vi "sensitivity (yzb).vi"(7 "sense":bool, 8 "error in (no error)":errorcluster, 11 "VISA resource name":refnum<visa-resource-name>="GPIB0::8::INSTR") -> (0 "error out":errorcluster, 5 "Sensitivity":i16(ring)=-1 items=["Auto Gain"=-1, "2 nV/fA"=0, "5 nV/fA"=1, "10 nV/fA"=2, "20 nV/fA"=3, "50 nV/fA"=4, "100 nV/fA"=5, "200 nV/fA"=6, "500 nV/fA"=7, "1 uV/pA"=8, "2 uV/pA"=9, "5 uV/pA"=10, "10 uV/pA"=11, "20 uV/pA"=12, "50 uV/pA"=13, "100 uV/pA"=14, "200 uV/pA"=15, "500 uV/pA"=16, "1 mV/nA"=17, "2 mV/nA"=18, "5 mV/nA"=19, "10 mV/nA"=20, "20 mV/nA"=21, "50 mV/nA"=22, "100 mV/nA"=23, "200 mV/nA"=24, "500 mV/mA"=25, "1 V/uA"=26])   [LabVIEW 2017]
uses:
  <vilib>/Analysis/NI_AALBase.lvlib
panel:
  out "Array":dbl[](array[numeric])
  out "Numeric":i32
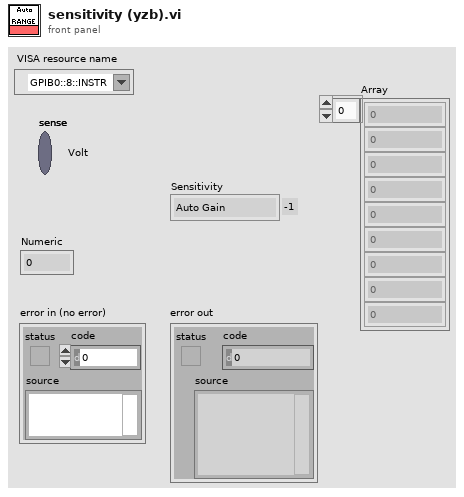
[diagram p1: front panel]
types:
  T1 = cluster{"X-Value":dbl, "Y-Value":dbl, "R-Value":dbl, "Theta-Value":dbl, "Channel 1 Display":dbl, "Channel 2 Display":dbl}
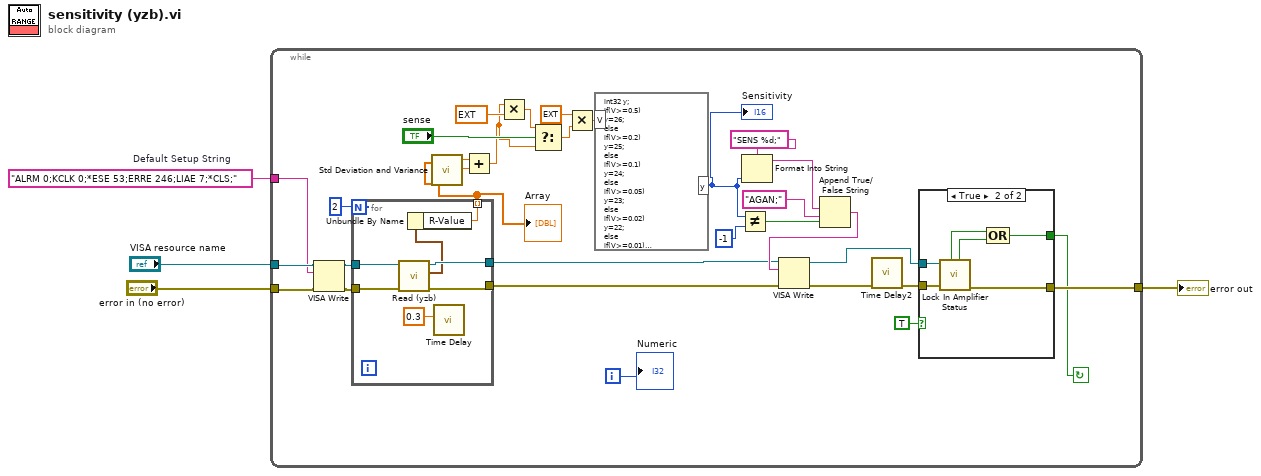
[diagram p0: block diagram]
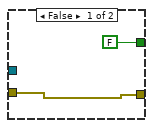
[diagram p2: hidden frame]
diagram:
  w2 = "ALRM 0;KCLK 0;*ESE 53;ERRE 246;LIAE 7;*CLS;"  # Default Setup String
  n1 = while {
    tunnel: "VISA resource name" -> [w24]
    tunnel: [w27] -> w1
    tunnel: "error in (no error)" -> [w26]
    tunnel: w2 -> [w22]
    i -> [w36]
    stop <- w17 continue-if-true
    n2 = VISA Write(VISA resource name=w24, write buffer=w22, error in (no error)=w26) -> (VISA resource name out=w23:refnum<visa-resource-name>, error out=w25:errorcluster)  [unwired: 1 out]
    n3 = for {
      N: 2 -> [_]
      tunnel: w23 -> [w51]
      tunnel: w25 -> [w50]
      tunnel: [w48] -> w19
      tunnel: [w49] -> w8 mode=indexing
      tunnel: [w46] -> w18
      n4 = call "Read (yzb).vi"("error in (no error)"=w50, "VISA resource name"=w51) -> ("error out"=w46:errorcluster, "Parameter Values"=w47:T1, "VISA resource name out"=w48:refnum<visa-resource-name>)  [unwired: 7 in]
      n5 = Unbundle By Name(w47) -> ("R-Value"=w49:dbl)
      n6 = call "Time Delay"("Delay Time (s)"=0.3) -> ()  [unwired: 10 in, 1 out]
    }
    "Array" <- w8
    n7 = call <vilib>:"Std Deviation and Variance.vi"("X"=w8) -> ("mean"=w7:dbl, "standard deviation"=w6:dbl)  [unwired: 1 in, 1 out]
    n8 = Add(x=w7, y=w6) -> (x+y=w5:dbl)
    n9 = Multiply(x=w5, y=ext 1000000.0) -> (x*y=w14:ext)
    n10 = Select(t=w14, s="sense", f=w5) -> (s? t:f=w12:ext)
    n11 = Multiply(x=ext 1.1, y=w12) -> (x*y=w10:ext)
    n12 = formula code="int32 y;\nif(V>=0.5)\ny=26;\nelse\nif(V>=0.2)\ny=25;\nelse\nif(V>=0.1)\ny=24;\nelse\nif(V>=0.05)\ny=23;\nelse\nif(V>=0.02)\ny=22;\nelse\nif(V>=0.01)\ny=21;\nelse\nif(V>=0.005)\ny=20;\nelse\nif(V>=0.002)\ny=19;\nelse\nif(V>=0.001)\ny=18;\nelse\nif(V>=0.0005)\ny=17;\nelse\nif(V>=0.0002)\ny=16;\nelse\nif(V>=0.0001)\ny=15;\nelse\nif(V>=0.00005)\ny=14;\nelse\nif(V>=0.00002)\ny=13;\nelse\nif (V>=0.00001)\ny=12;\nelse\nif(V>=0.000005)\ny=11;\nelse\nif(V>=0.000002)\ny=10;\nelse\nif(V>=0.000001)\ny=9;\nelse\nif(V>=0.0000005)\ny=8;\nelse\nif(V>=0.0000002)\ny=7;\nelse\nif(V>=0.0000001)\ny=6;\nelse\nif(V>=0.00000005)\ny=5;\nelse\nif(V>=0.00000002)\ny=4;\nelse\nif(V>=0.00000001)\ny=3;\nelse\nif(V>=0.000000005)\ny=2;\nelse\nif(V>=0.000000005)\ny=1;\nelse\ny=1;"("V"=w10) -> ("y"=w13:i32)
    "Sensitivity" <- w13
    n13 = Not Equal?(x=w13, y=i16 -1) -> (x != y?=w34:bool)
    n14 = Format Into String(format string="SENS %d;", w13) -> (resulting string=w33:string)  [unwired: 2 in, 1 out]
    n15 = Append True/False String(1:w34, 2:"AGAN;" ("false string"), 3:w33) -> (0:w29:string)  [unwired: 1 in]
    n16 = VISA Write(VISA resource name=w19, write buffer=w29, error in (no error)=w18) -> (VISA resource name out=w28:refnum<visa-resource-name>, error out=w21:errorcluster)  [unwired: 1 out]
    n17 = call "Time Delay2"("error in (no error)"=w21) -> ("error out"=w20:errorcluster)  [unwired: 10 in]
    n18 = case shown="True" TRUE {
      tunnel: w28 -> [_ w44]
      tunnel: [w38 w43] -> w27
      tunnel: w20 -> [w38 w42]
      tunnel: [FALSE w39] -> w17
      frame False {
      }
      frame True {
        n19 = call "Lock In Amplifier Status.vi"("error in (no error)"=w42, "VISA resource name"=w44) -> ("error out"=w43:errorcluster, "Time overload"=w40:bool, "output overload"=w41:bool)  [unwired: 4 in, 3 out]
        n20 = Compound Arithmetic op=OR(w41, w40) -> (w39:bool)
      }
    }
    "Numeric" <- w36
  }
  "error out" <- w1
